vi "tag_open_subvi.vi"() -> (8 "error out":errorcluster, 9 "STOPWEB":refnum<class "NI Skyline Tag.lvclass">, 14 "User-T":refnum<class "NI Skyline Tag.lvclass">, 15 "Coffee-T":refnum<class "NI Skyline Tag.lvclass">, 16 "Plate-T":refnum<class "NI Skyline Tag.lvclass">, 17 "Hot-Sfc":refnum<class "NI Skyline Tag.lvclass">, 18 "Plate-ON":refnum<class "NI Skyline Tag.lvclass">, 19 "Warn String":refnum<class "NI Skyline Tag.lvclass">)   [LabVIEW 2021]
uses:
  <vilib>/Skyline/Tag/Wrapper/Wrapper_class/NI Skyline Tag.lvclass
  <vilib>/Skyline/Tag/Shared/typedefs/DataType.ctl
  <vilib>/Skyline/Configuration/Configuration HTTP_class/Open Configuration API Key.vi
  <vilib>/Skyline/Configuration/Configuration HTTP_class/NI Skyline Configuration HTTP.lvclass
  <vilib>/Skyline/Tag/Wrapper/Wrapper HTTP_class/NI Skyline Tag HTTP.lvclass
  <vilib>/Skyline/Tag/Shared/NI Skyline Tag.lvlib
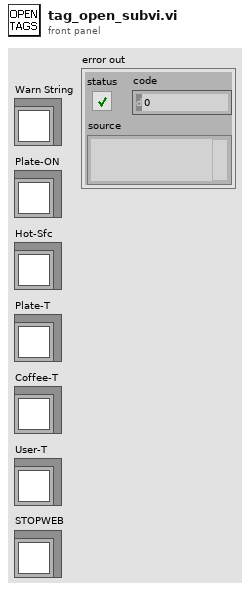
[diagram p1: front panel]
types:
  T1 = typedef "NI Skyline Tag.lvlib/DataType.ctl" = enum32{"Double", "I32", "String", "Boolean", "U64", "Timestamp"}
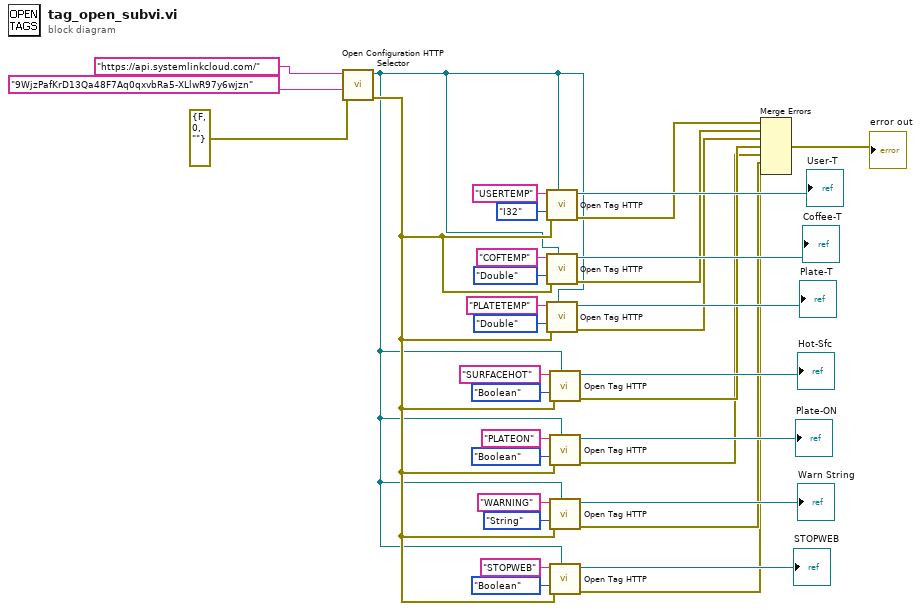
[diagram p0: block diagram]
diagram:
  n1 = call-poly <vilib>:"Open Configuration HTTP Selector.vi"("error in (no error)"=errorcluster {"status"=FALSE, "code"=0, "source"=""}, "api key"="9WjzPafKrD13Qa48F7Aq0qxvbRa5-XLlwR97y6wjzn" ("username"), "server url"="https://api.systemlinkcloud.com/") -> ("error out"=w12:errorcluster, "configuration"=w2:refnum<class "NI Skyline Configuration HTTP.lvclass">)  [unwired: 7 in]
  n2 = call <vilib>:"Open Tag HTTP.vi"("configuration"=w2, "error in (no error)"=w12, "Data Type"=DataType."I32", "path"="USERTEMP") -> ("error out"=w9:errorcluster, "tag"=→"User-T":refnum<class "NI Skyline Tag.lvclass">)  [unwired: 6 in]
  n3 = call <vilib>:"Open Tag HTTP.vi"("configuration"=w2, "error in (no error)"=w12, "Data Type"=DataType."Double", "path"="COFTEMP") -> ("error out"=w8:errorcluster, "tag"=→"Coffee-T":refnum<class "NI Skyline Tag.lvclass">)  [unwired: 6 in]
  n4 = call <vilib>:"Open Tag HTTP.vi"("configuration"=w2, "error in (no error)"=w12, "Data Type"=DataType."Double", "path"="PLATETEMP") -> ("error out"=w7:errorcluster, "tag"=→"Plate-T":refnum<class "NI Skyline Tag.lvclass">)  [unwired: 6 in]
  n5 = call <vilib>:"Open Tag HTTP.vi"("configuration"=w2, "error in (no error)"=w12, "Data Type"=DataType."Boolean", "path"="SURFACEHOT") -> ("error out"=w6:errorcluster, "tag"=→"Hot-Sfc":refnum<class "NI Skyline Tag.lvclass">)  [unwired: 6 in]
  n6 = call <vilib>:"Open Tag HTTP.vi"("configuration"=w2, "error in (no error)"=w12, "Data Type"=DataType."Boolean", "path"="PLATEON") -> ("error out"=w5:errorcluster, "tag"=→"Plate-ON":refnum<class "NI Skyline Tag.lvclass">)  [unwired: 6 in]
  n7 = call <vilib>:"Open Tag HTTP.vi"("configuration"=w2, "error in (no error)"=w12, "Data Type"=DataType."String", "path"="WARNING") -> ("error out"=w4:errorcluster, "tag"=→"Warn String":refnum<class "NI Skyline Tag.lvclass">)  [unwired: 6 in]
  n8 = call <vilib>:"Open Tag HTTP.vi"("configuration"=w2, "error in (no error)"=w12, "Data Type"=DataType."Boolean", "path"="STOPWEB") -> ("error out"=w3:errorcluster, "tag"=→"STOPWEB":refnum<class "NI Skyline Tag.lvclass">)  [unwired: 6 in]
  n9 = Merge Errors(w9, w8, w7, w6, w5, w4, w3) -> (→"error out":errorcluster)
